vi "HEWH Check Ambient Temp.vi"(7 "Water Heater Type":T1, 8 "error in (no error)":errorcluster, 11 "UEF Calculated Values Input":T2 {"Data Indexes"."15 sec after Draw Index" format="%#.2f"; "Data Indexes"."15 sec after Draw Timestamp" format="%#.2f"; "Data Indexes"."Test Start Timestamp" format="%.2f"; "Data Indexes"."Test End Timestamp" format="%.2f"; "Data Indexes"."T0 Timestamp" format="%.2f"; "Data Indexes"."Tsf Timestamp" format="%.2f"; "Data Indexes"."Tsu0 Timestamp" format="%.2f"; "Data Indexes"."Tmax1 Timestamp" format="%.2f"; "Data Indexes"."Draw Index Timestamp" format="%#.2f"; "Data Indexes"."Non-Draw Timestamp" format="%#.2f"; "Data Indexes"."Heating Timestamp" format="%#.2f"; "Data Indexes"."Start Energy (BTU-Gas)" format="%.6f"; "Data Indexes"."Start Watt Hours" format="%.6f"; "Static Data"."V - Volume of Wh (True)" format="%.5f"; "Static Data"."T-Ambinet Nominal (°F)" format="%.5f"; "Static Data"."T-Inlet Setpoint (°F)" format="%.5f"; "Static Data"."T-Wh Setpoint (°F)" format="%.5f"; "Sampled Data"."Qe (Wh)" format="%.5f"; "Sampled Data"."Tau stby2 (hr)" format="%.5f"; "Sampled Data"."Tastby2 (°F)" format="%.5f"; "Sampled Data"."Qf (BTU)" format="%.5f"; "Sampled Data"."Qe (BTU)" format="%.5f"; "Sampled Data"."Tmax1 (°F)" format="%.5f"; "Sampled Data"."T0 (°F)" format="%.5f"; "Sampled Data"."Qr (BTU)" format="%.5f"; "Sampled Data"."T 24(°F)" format="%.5f"; "Sampled Data"."T astby(°F)" format="%.5f"; "Sampled Data"."T tstby(°F)" format="%.5f"; "Sampled Data"."T su0(°F)" format="%.5f"; "Sampled Data"."T suf(°F)" format="%.5f"; "Sampled Data"."Tau stby_1 (hr)" format="%.5f"; "Sampled Data"."Qsuf (BTU)" format="%.5f"; "Sampled Data"."Qsu0 (BTU)" format="%.5f"; "Calculated Values"."Draw Bonus Volume (gal)" format="%.6f"; "Calculated Values"."Adjustment Factor" format="%.6f"; "Calculated Values"."T*avg_del(n-1)" format="%.6f"; "Calculated Values"."T*min(n-1)" format="%.6f"; "Calculated Values"."T*avg_del(n)" format="%.6f"; "Calculated Values"."Vn" format="%.6f"; "Calculated Values"."Qdm (BTU)" format="%.6f"; "Calculated Values"."QHWD (BTU)" format="%.6f"; "Calculated Values"."QHW (BTU)" format="%.6f"; "Calculated Values"."UEF" format="%.6f"; "Calculated Values"."QHW67 (BTU)" format="%.6f"; "Calculated Values"."Qda (BTU)" format="%.6f"; "Calculated Values"."Qd (BTU)" format="%.6f"; "Calculated Values"."Q (BTU)" format="%.6f"; "Calculated Values"."UA (BTU/(hr*F))" format="%.6f"; "Calculated Values"."Qhr (BTU/hr)" format="%.6f"; "Calculated Values"."Qstby (BTU)" format="%.6f"; "Calculated Values"."nu_r" format="%.6f"; "Calculated Values"."CpUEF (BTU/(lb*F))" format="%.6f"; "Calculated Values"."rho_nu (lb/gal)" format="%.6f"; "Calculated Values"."V1- Vol (Gal)" format="%.6f"; "Calculated Values"."M cluster mass removed (lb)" format="%.6f"; "Calculated Values"."Cp theoretical (BTU/(lbm °F))" format="%.6f"; "Calculated Values"."Tin1 - Mean Inlet 1st Cluster (°F)" format="%.6f"; "Calculated Values"."Tdel1-Mean Outlet 1st Cluster(°F)" format="%.6f"; "Calculated Values"."Cp 24 (BTU/(lb*F))" format="%.6f"; "Calculated Values"."Cp standby (BTU/(lb*F))" format="%.6f"; "Calculated Values"."Cp2 (BTU/(lb*F))" format="%.6f"; "Calculated Values"."Cp1 (BTU/(lb*F))" format="%.6f"; "Calculated Values"."rho 24 (lb/gal)" format="%.6f"; "Calculated Values"."rho standby (lb/gal)" format="%.6f"; "Calculated Values"."rho 2 (lb/gal)" format="%.6f"; "Calculated Values"."Density of cold water All (lbm/gal)" format="%#.3g"; "Calculated Values"."CpHW (BTU/(lbm °F))" format="%#.3g"; "Calculated Values"."Density of hot water All (lbm/gal)" format="%#.3g"; "Calculated Values"."Mass of water All (lbm)" format="%#.3f"}) -> (0 "error out":errorcluster, 3 "UEF Calculated Values Output":T2 {"Data Indexes"."15 sec after Draw Index" format="%#.2f"; "Data Indexes"."15 sec after Draw Timestamp" format="%#.2f"; "Data Indexes"."Test Start Timestamp" format="%.2f"; "Data Indexes"."Test End Timestamp" format="%.2f"; "Data Indexes"."T0 Timestamp" format="%.2f"; "Data Indexes"."Tsf Timestamp" format="%.2f"; "Data Indexes"."Tsu0 Timestamp" format="%.2f"; "Data Indexes"."Tmax1 Timestamp" format="%.2f"; "Data Indexes"."Draw Index Timestamp" format="%#.2f"; "Data Indexes"."Non-Draw Timestamp" format="%#.2f"; "Data Indexes"."Heating Timestamp" format="%#.2f"; "Data Indexes"."Start Energy (BTU-Gas)" format="%.6f"; "Data Indexes"."Start Watt Hours" format="%.6f"; "Static Data"."V - Volume of Wh (True)" format="%.5f"; "Static Data"."T-Ambinet Nominal (°F)" format="%.5f"; "Static Data"."T-Inlet Setpoint (°F)" format="%.5f"; "Static Data"."T-Wh Setpoint (°F)" format="%.5f"; "Sampled Data"."Qe (Wh)" format="%.5f"; "Sampled Data"."Tau stby2 (hr)" format="%.5f"; "Sampled Data"."Tastby2 (°F)" format="%.5f"; "Sampled Data"."Qf (BTU)" format="%.5f"; "Sampled Data"."Qe (BTU)" format="%.5f"; "Sampled Data"."Tmax1 (°F)" format="%.5f"; "Sampled Data"."T0 (°F)" format="%.5f"; "Sampled Data"."Qr (BTU)" format="%.5f"; "Sampled Data"."T 24(°F)" format="%.5f"; "Sampled Data"."T astby(°F)" format="%.5f"; "Sampled Data"."T tstby(°F)" format="%.5f"; "Sampled Data"."T su0(°F)" format="%.5f"; "Sampled Data"."T suf(°F)" format="%.5f"; "Sampled Data"."Tau stby_1 (hr)" format="%.5f"; "Sampled Data"."Qsuf (BTU)" format="%.5f"; "Sampled Data"."Qsu0 (BTU)" format="%.5f"; "Calculated Values"."Draw Bonus Volume (gal)" format="%.6f"; "Calculated Values"."Adjustment Factor" format="%.6f"; "Calculated Values"."T*avg_del(n-1)" format="%.6f"; "Calculated Values"."T*min(n-1)" format="%.6f"; "Calculated Values"."T*avg_del(n)" format="%.6f"; "Calculated Values"."Vn" format="%.6f"; "Calculated Values"."Qdm (BTU)" format="%.6f"; "Calculated Values"."QHWD (BTU)" format="%.6f"; "Calculated Values"."QHW (BTU)" format="%.6f"; "Calculated Values"."UEF" format="%.6f"; "Calculated Values"."QHW67 (BTU)" format="%.6f"; "Calculated Values"."Qda (BTU)" format="%.6f"; "Calculated Values"."Qd (BTU)" format="%.6f"; "Calculated Values"."Q (BTU)" format="%.6f"; "Calculated Values"."UA (BTU/(hr*F))" format="%.6f"; "Calculated Values"."Qhr (BTU/hr)" format="%.6f"; "Calculated Values"."Qstby (BTU)" format="%.6f"; "Calculated Values"."nu_r" format="%.6f"; "Calculated Values"."CpUEF (BTU/(lb*F))" format="%.6f"; "Calculated Values"."rho_nu (lb/gal)" format="%.6f"; "Calculated Values"."V1- Vol (Gal)" format="%.6f"; "Calculated Values"."M cluster mass removed (lb)" format="%.6f"; "Calculated Values"."Cp theoretical (BTU/(lbm °F))" format="%.6f"; "Calculated Values"."Tin1 - Mean Inlet 1st Cluster (°F)" format="%.6f"; "Calculated Values"."Tdel1-Mean Outlet 1st Cluster(°F)" format="%.6f"; "Calculated Values"."Cp 24 (BTU/(lb*F))" format="%.6f"; "Calculated Values"."Cp standby (BTU/(lb*F))" format="%.6f"; "Calculated Values"."Cp2 (BTU/(lb*F))" format="%.6f"; "Calculated Values"."Cp1 (BTU/(lb*F))" format="%.6f"; "Calculated Values"."rho 24 (lb/gal)" format="%.6f"; "Calculated Values"."rho standby (lb/gal)" format="%.6f"; "Calculated Values"."rho 2 (lb/gal)" format="%.6f"; "Calculated Values"."Density of cold water All (lbm/gal)" format="%#.3g"; "Calculated Values"."CpHW (BTU/(lbm °F))" format="%#.3g"; "Calculated Values"."Density of hot water All (lbm/gal)" format="%#.3g"; "Calculated Values"."Mass of water All (lbm)" format="%#.3f"})   [LabVIEW 2023]
uses:
  Type Definitions/UEF Constants.ctl
  Type Definitions/HEWH Draw Stats.ctl
  Type Definitions/HEWH FHR Draw Type.ctl
  Type Definitions/FHR Bins.ctl
  Type Definitions/HEWH Meter Type.ctl
  Type Definitions/HEWH Water Heater Type.ctl
panel:
  # "FHR"
  # "FHR"
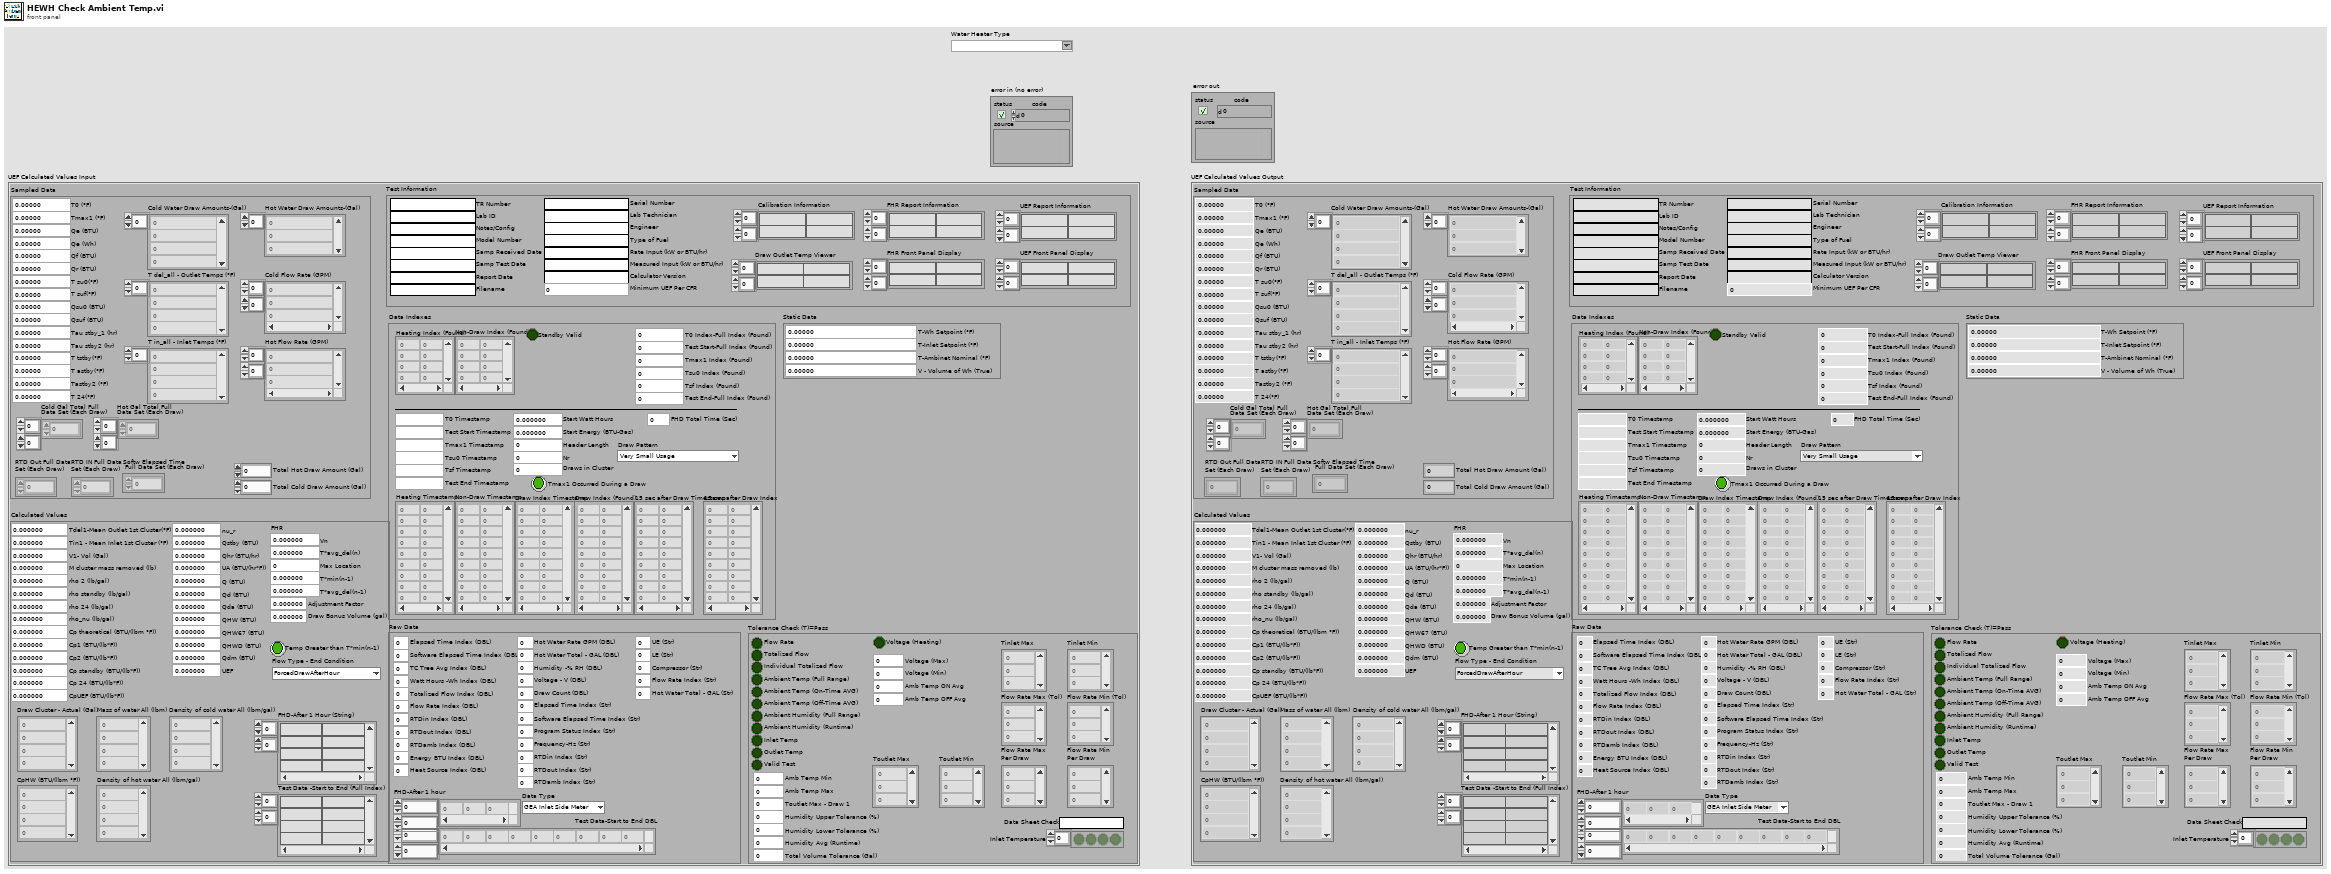
[diagram p1: front panel]
types:
  T1 = typedef "HEWH Water Heater Type.ctl" = string
  T2 = typedef "UEF Constants.ctl" = cluster{"Calculated Values":T3, "Sampled Data":cluster{"Cold Water Draw Amounts-(Gal)":dbl[], "T del_all - Outlet Temps (°F)":dbl[], "T in_all - Inlet Temps (°F)":dbl[], "Qsu0 (BTU)":dbl, "Qsuf (BTU)":dbl, "Tau stby_1 (hr)":dbl, "T suf(°F)":dbl, "T su0(°F)":dbl, "T tstby(°F)":dbl, "T astby(°F)":dbl, "T 24(°F)":dbl, "Qr (BTU)":dbl, "T0 (°F)":dbl, "Tmax1 (°F)":dbl, "Qe (BTU)":dbl, "Qf (BTU)":dbl, "Tastby2 (°F)":dbl, "RTD Out Full Data\nSet (Each Draw)":dbl[][], "RTD IN Full Data\nSet (Each Draw)":dbl[][], "Tau stby2 (hr)":dbl, "Hot Water Draw Amounts-(Gal)":dbl[], "Cold Flow Rate (GPM)":dbl[][], "Hot Flow Rate (GPM)":dbl[][], "Softw Elapsed Time\n Full Data Set (Each Draw)":dbl[][], "Cold Gal Total Full\nData Set (Each Draw)":dbl[][], "Total Hot Draw Amount (Gal) ":dbl, "Total Cold Draw Amount (Gal)":dbl, "Qe (Wh)":dbl, "Hot Gal Total Full\nData Set (Each Draw)":dbl[][]}, "Static Data":cluster{"T-Wh Setpoint (°F)":dbl, "T-Inlet Setpoint (°F)":dbl, "T-Ambinet Nominal (°F)":dbl, "V - Volume of Wh (True)":dbl}, "Data Indexes":cluster{"Test Start-Full Index (Found)":i32, "Header Length":i32, "Draw Index (Found)":i32[][], "Nr":i32, "Start Watt Hours":dbl, "Tsu0 Index (Found)":i32, "Tsf Index (Found)":i32, "Start Energy (BTU-Gas)":dbl, "Draws in Cluster":i32, "T0 Index-Full Index (Found)":i32, "Non-Draw Index (Found)":i32[][], "Tmax1 Index (Found)":i32, "Test End-Full Index (Found)":i32, "Heating Index (Found)":i32[][], "Heating Timestamp":dbl[][], "Non-Draw Timestamp":dbl[][], "Draw Index Timestamp":dbl[][], "Tmax1 Timestamp":dbl, "Tsu0 Timestamp":dbl, "Tsf Timestamp":dbl, "T0 Timestamp":dbl, "Test End Timestamp":dbl, "Test Start Timestamp":dbl, "15 sec after Draw Timestamp":dbl[][], "15 sec after Draw Index":dbl[][], "Tmax1 Occurred During a Draw":bool, "FHD Total Time (Sec)":dbl, "Draw Pattern":T5, "Standby Valid":bool}, "Raw Data":cluster{"Elapsed Time Index (DBL)":i32, "Software Elapsed Time Index (DBL)":i32, "TC Tree Avg Index (DBL)":i32, "Watt Hours -Wh Index (DBL)":i32, "Energy BTU Index (DBL)":i32, "Totalized Flow Index (DBL)":i32, "Flow Rate Index (DBL)":i32, "Program Status Index (Str)":i32, "RTDin Index (DBL)":i32, "RTDout Index (DBL)":i32, "RTDamb Index (DBL)":i32, "Test Data-Start to End DBL":dbl[][], "Data Type":T6, "Heat Source Index (DBL)":i32, "Hot Water Rate GPM (DBL)":i32, "Hot Water Total - GAL (DBL)":i32, "FHD-After 1 hour":dbl[][], "Humidity -% RH (DBL)":i32, "Voltage - V (DBL)":i32, "Draw Count (DBL)":i32, "Elapsed Time Index (Str)":i32, "Software Elapsed Time Index (Str)":i32, "Frequency-Hz (Str)":i32, "RTDin Index (Str)":i32, "RTDout Index (Str)":i32, "RTDamb Index (Str)":i32, "UE (Str)":i32, "LE (Str)":i32, "Compressor (Str)":i32, "Flow Rate Index (Str)":i32, "Hot Water Total - GAL (Str)":i32}, "Tolerance Check (T)=Pass":cluster{"Flow Rate":bool, "Totalized Flow":bool, "Ambient Temp (Full Range)":bool, "Ambient Humidity (Full Range)":bool, "Inlet Temp":bool, "Outlet Temp":bool, "Valid Test":bool, "Individual Totalized Flow":bool, "Data Sheet Check":string, "Inlet Temperature":bool[], "Tinlet Max":dbl[], "Tinlet Min":dbl[], "Flow Rate Max (Tol)":dbl[], "Flow Rate Min (Tol)":dbl[], "Amb Temp Max":dbl, "Amb Temp Min":dbl, "Toutlet Max - Draw 1":dbl, "Humidity Upper Tolerance (%)":dbl, "Total Volume Tolerance (Gal)":dbl, "Humidity Lower Tolerance (%)":dbl, "Flow Rate Max\nPer Draw":dbl[], "Flow Rate Min\nPer Draw":dbl[], "Ambient Humidity (Runtime)":bool, "Humidity Avg (Runtime)":dbl, "Ambient Temp (On-Time AVG)":bool, "Ambient Temp (Off-Time AVG)":bool, "Amb Temp OFF Avg":dbl, "Amb Temp ON Avg":dbl, "Voltage (Heating)":bool, "Voltage (Min)":dbl, "Voltage (Max)":dbl, "Toutlet Max":dbl[], "Toutlet Min":dbl[]}, "Test Information":cluster{"TR Number":string, "Lab ID":string, "Notes/Config":string, "Model Number":string, "Serial Number":string, "Lab Technician":string, "Engineer":string, "Type of Fuel":string, "Samp Received Date":string, "Samp Test Date":string, "Report Date":string, "Rate Input (kW or BTU/hr)":string, "Measured Input (kW or BTU/hr)":string, "Filename":string, "Calibration Information":string[][], "Calculator Version":string, "Minimum UEF Per CFR":dbl, "UEF Report Information":string[][], "FHR Report Information":string[][], "FHR Front Panel Display":string[][], "UEF Front Panel Display":string[][], "Draw Outlet Temp Viewer":string[][]}}
  T3 = typedef "HEWH Draw Stats.ctl" = cluster{"Draw Cluster - Actual (Gal)":dbl[], "Mass of water All (lbm)":dbl[], "Density of hot water All (lbm/gal)":dbl[], "CpHW (BTU/(lbm °F))":dbl[], "rho 2 (lb/gal)":dbl, "rho standby (lb/gal)":dbl, "rho 24 (lb/gal)":dbl, "Cp1 (BTU/(lb*F))":dbl, "Cp2 (BTU/(lb*F))":dbl, "Cp standby (BTU/(lb*F))":dbl, "Cp 24 (BTU/(lb*F))":dbl, "nu_r":dbl, "Qstby (BTU)":dbl, "Qhr (BTU/hr)":dbl, "UA (BTU/(hr*F))":dbl, "Q (BTU)":dbl, "Qd (BTU)":dbl, "Qda (BTU)":dbl, "QHW67 (BTU)":dbl, "UEF":dbl, "Tdel1-Mean Outlet 1st Cluster(°F)":dbl, "Tin1 - Mean Inlet 1st Cluster (°F)":dbl, "Cp theoretical (BTU/(lbm °F))":dbl, "M cluster mass removed (lb)":dbl, "V1- Vol (Gal)":dbl, "Test Data -Start to End (Full Index)":string[][], "rho_nu (lb/gal)":dbl, "Density of cold water All (lbm/gal)":dbl[], "CpUEF (BTU/(lb*F))":dbl, "QHW (BTU)":dbl, "QHWD (BTU)":dbl, "Qdm (BTU)":dbl, "FHD-After 1 Hour (String)":string[][], "Vn":dbl, "T*avg_del(n)":dbl, "Max Location":i32, "T*min(n-1)":dbl, "T*avg_del(n-1)":dbl, "Temp Greater than T*min(n-1)":bool, "Adjustment Factor":dbl, "Draw Bonus Volume (gal)":dbl, "Flow Type - End Condition":T4}
  T4 = typedef "HEWH FHR Draw Type.ctl" = enum16{"ForcedDrawAfterHour", "HeatingCutoffBeforeHour"}
  T5 = typedef "FHR Bins.ctl" = enum16{"Very Small Usage", "Low Usage", "Medium Usage", "High Usage", "Undefined"}
  T6 = typedef "HEWH Meter Type.ctl" = enum16{"GEA Inlet Side Meter", "GEA Outlet Side Meter", "CSA Inlet Side Meter"}
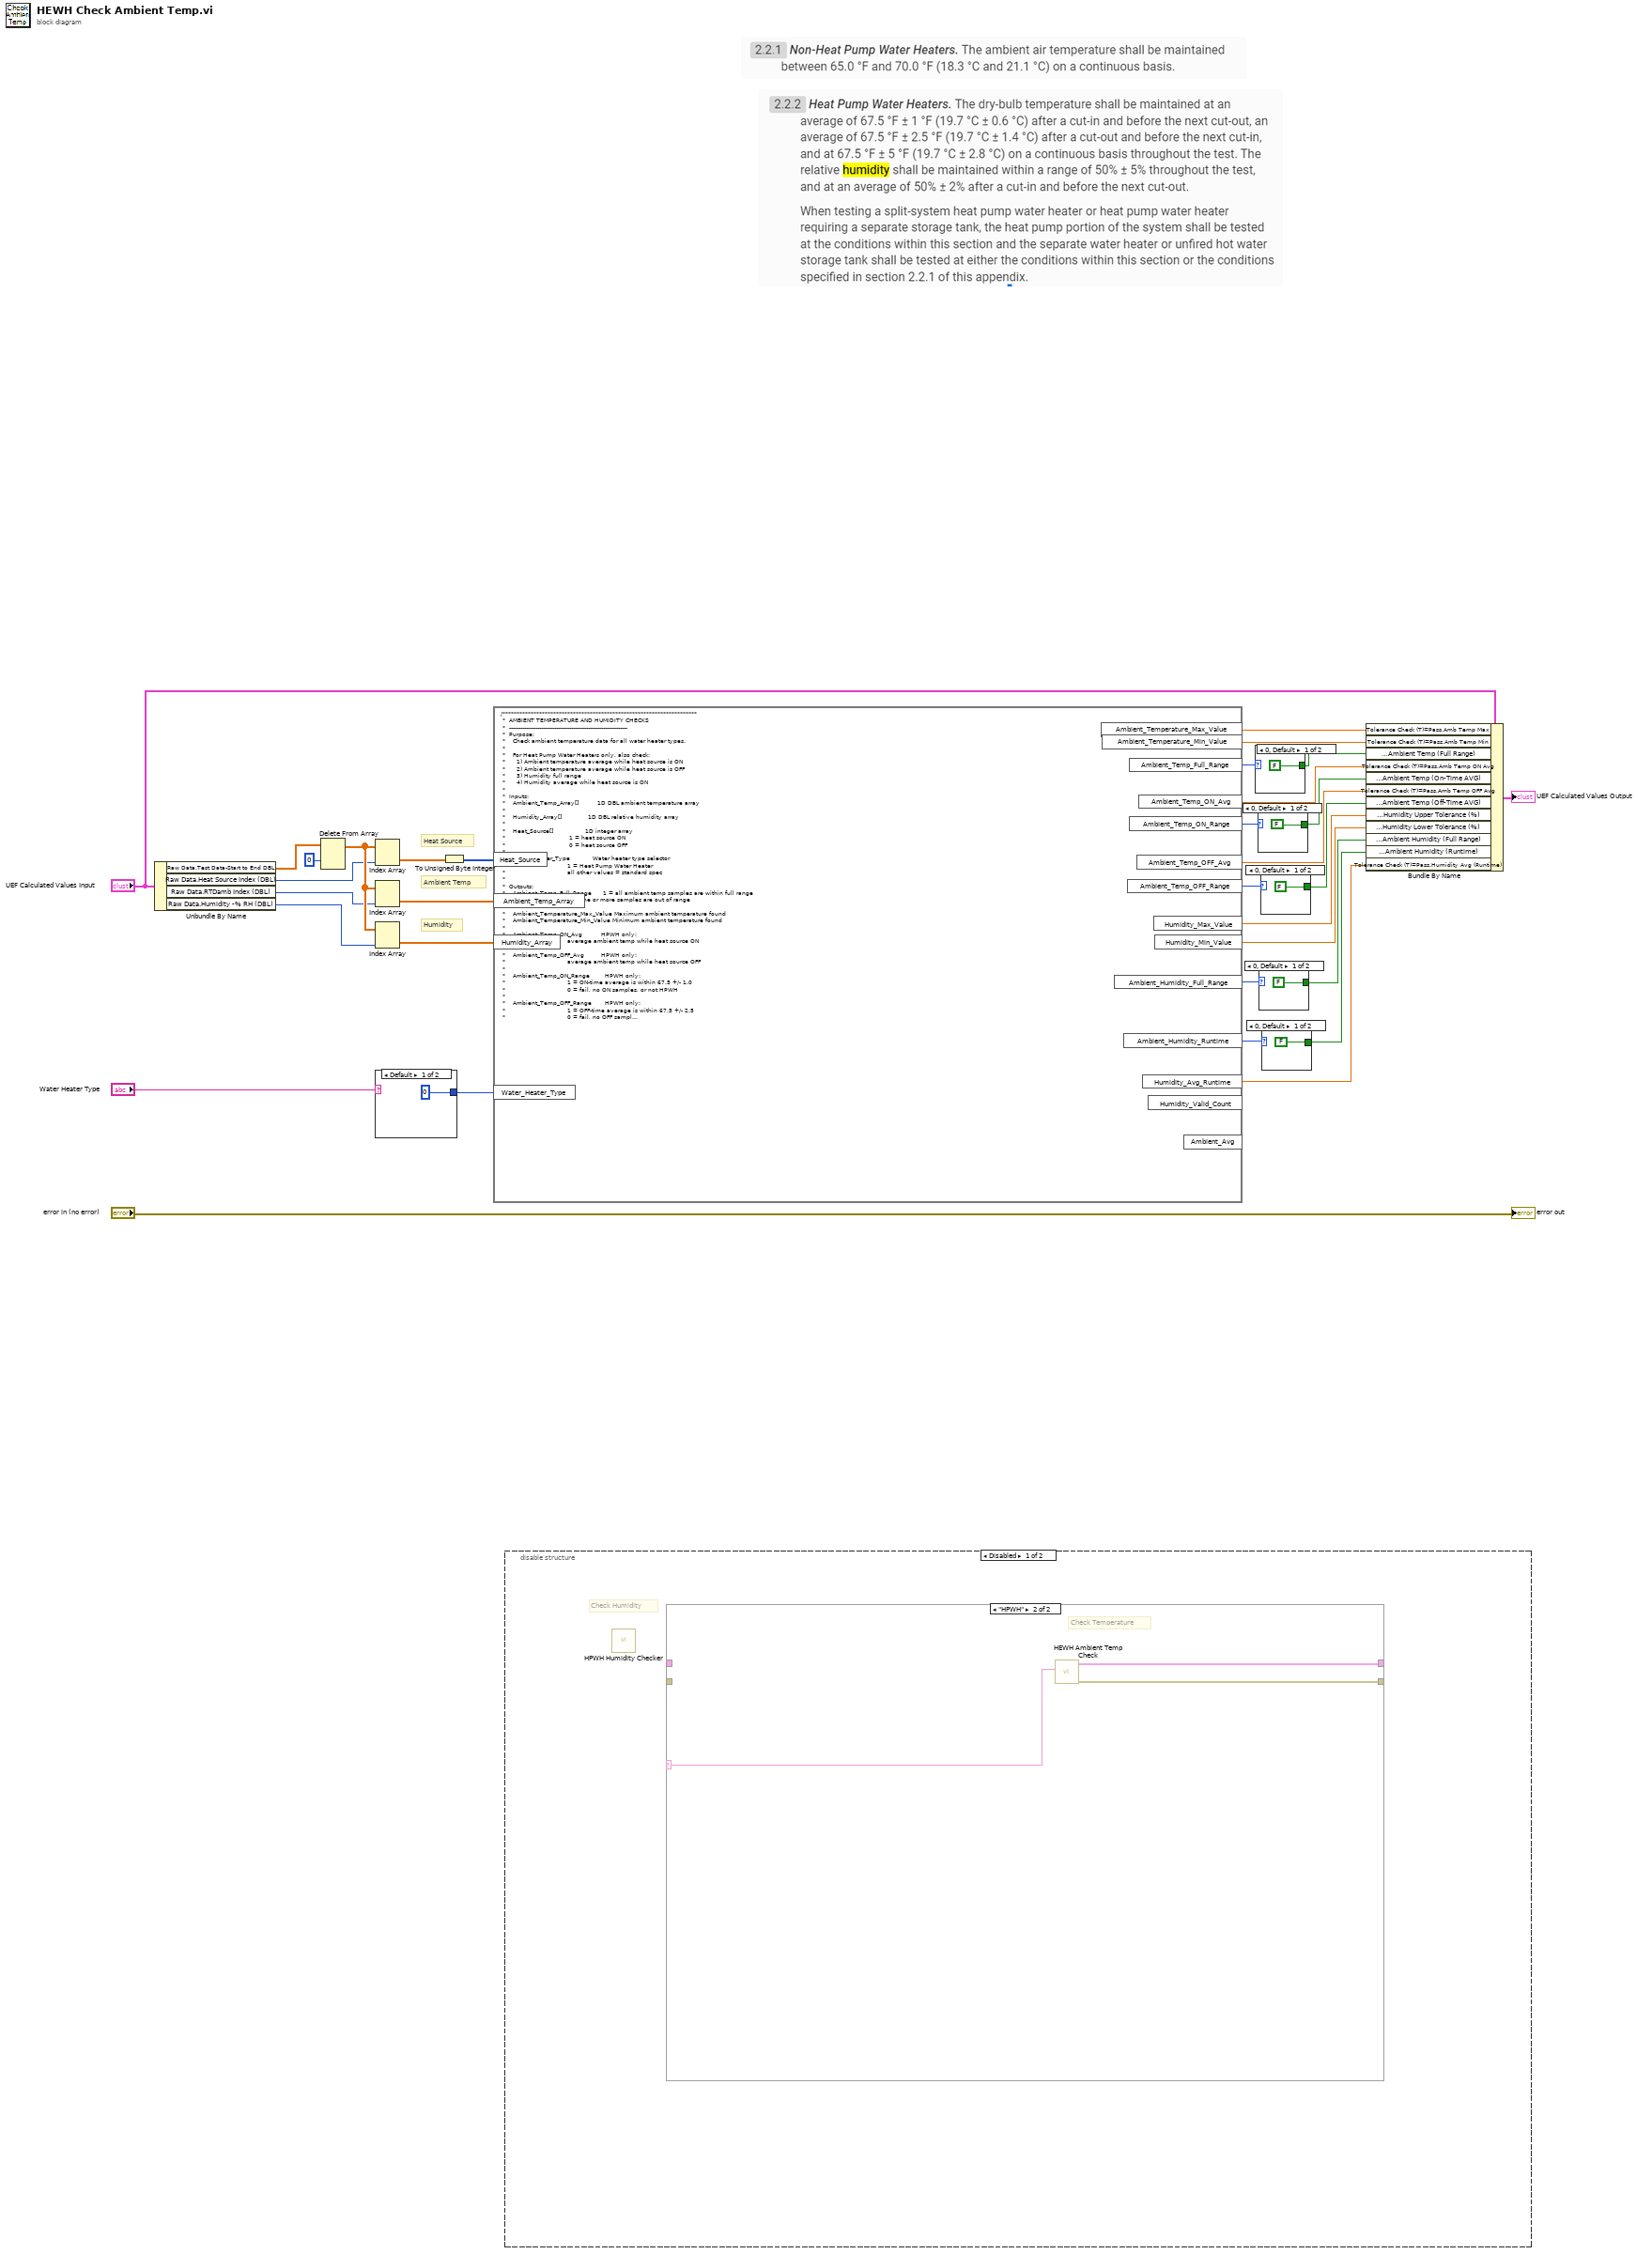
[diagram p0: block diagram]
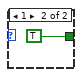
[diagram p2: hidden frame]
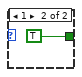
[diagram p3: hidden frame]
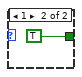
[diagram p4: hidden frame]
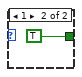
[diagram p5: hidden frame]
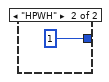
[diagram p6: hidden frame]
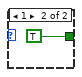
[diagram p7: hidden frame]
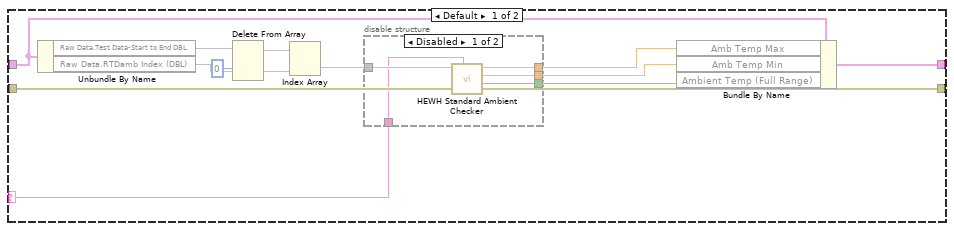
[diagram p8: hidden frame]
diagram:
  # "Humidity"
  # "Ambient Temp"
  # "Heat Source"
  n1 = Unbundle By Name("UEF Calculated Values Input") -> ("Raw Data.Test Data-Start to End DBL"=w9:dbl[][], "Raw Data.Heat Source Index (DBL)"=w7:i32, "Raw Data.RTDamb Index (DBL)"=w8:i32, "Raw Data.Humidity -% RH (DBL)"=w19:i32)
  n2 = Delete From Array(array=w9, index (row)=0) -> (array with subset deleted=w18:dbl[][])  [unwired: 2 in, 1 out]
  n3 = Index Array(array=w18, index (col)=w7) -> (element=w10:dbl[])  [unwired: 1 in]
  n4 = Index Array(array=w18, index (col)=w8) -> (element=w13:dbl[])  [unwired: 1 in]
  n5 = Index Array(array=w18, index (col)=w19) -> (element=w1:dbl[])  [unwired: 1 in]
  n6 = case shown="Default" "Water Heater Type" {
    tunnel: [0 ("Water_Heater_Type") 1 ("Water_Heater_Type")] -> w11
    frame Default {
    }
    frame "HPWH" {
    }
  }
  n7 = To Unsigned Byte Integer(number=w10) -> (unsigned 8bit integer=w14:u8[])
  n8 = formula code="/*********************************************************************\n *  AMBIENT TEMPERATURE AND HUMIDITY CHECKS\n *  ---------------------------------------------------------------\n *  Purpose:\n *    Check ambient temperature data for all water heater types.\n *\n *    For Heat Pump Water Heaters only, also check:\n *      1) Ambient temperature average while heat source is ON\n *      2) Ambient temperature average while heat source is OFF\n *      3) Humidity full range\n *      4) Humidity average while heat source is ON\n *\n *  Inputs:\n *    Ambient_Temp_Array[]          1D DBL ambient temperature array\n *\n *    Humidity_Array[]              1D DBL relative humidity array\n *\n *    Heat_Source[]                 1D integer array\n *                                  1 = heat source ON\n *                                  0 = heat source OFF\n *\n *    Water_Heater_Type            Water heater type selector\n *                                 1 = Heat Pump Water Heater\n *                                 all other values = standard spec\n *\n *  Outputs:\n *    Ambient_Temp_Full_Range      1 = all ambient temp samples are within full range\n *                                 0 = one or more samples are out of range\n *\n *    Ambient_Temperature_Max_Value Maximum ambient temperature found\n *    Ambient_Temperature_Min_Value Minimum ambient temperature found\n *\n *    Ambient_Temp_ON_Avg          HPWH only:\n *                                 average ambient temp while heat source ON\n *\n *    Ambient_Temp_OFF_Avg         HPWH only:\n *                                 average ambient temp while heat source OFF\n *\n *    Ambient_Temp_ON_Range        HPWH only:\n *                                 1 = ON-time average is within 67.5 +/- 1.0\n *                                 0 = fail, no ON samples, or not HPWH\n *\n *    Ambient_Temp_OFF_Range       HPWH only:\n *                                 1 = OFF-time average is within 67.5 +/- 2.5\n *                                 0 = fail, no OFF samples, or not HPWH\n *\n *    Humidity_Max_Value           HPWH only:\n *                                 maximum humidity value found\n *\n *    Humidity_Min_Value           HPWH only:\n *                                 minimum humidity value found\n *\n *    Ambient_Humidity_Full_Range HPWH only:\n *                                 1 = full humidity array is within 50 +/- 5%\n *                                 0 = fail, empty array, or not HPWH\n *\n *    Humidity_Avg_Runtime         HPWH only:\n *                                 average humidity while heat source is ON\n *\n *    Ambient_Humidity_Runtime     HPWH only:\n *                                 1 = runtime humidity average is within 50 +/- 2%\n *                                 0 = fail, no ON samples, or not HPWH\n *\n *  Ambient Temperature Full Range Logic:\n *    Heat Pump Water Heater:\n *      Lower = 62.5\n *      Upper = 72.5\n *\n *    All other water heater types:\n *      Lower = 65.0\n *      Upper = 70.0\n *\n *  HPWH Ambient ON/OFF Average Logic:\n *    ON-time average:\n *      Lower = 66.5\n *      Upper = 68.5\n *\n *    OFF-time average:\n *      Lower = 65.0\n *      Upper = 70.0\n *\n *  HPWH Humidity Logic:\n *    Full-range humidity:\n *      Lower = 45.0\n *      Upper = 55.0\n *\n *    Runtime average humidity:\n *      Lower = 48.0\n *      Upper = 52.0\n *********************************************************************/\n\n\n/* ---------------- Local variables -------------------------------- */\n\nint32 i;\n\nint32 N;\nint32 N_Heat;\nint32 Loop_N;\n\nint32 ON_Count;\nint32 OFF_Count;\n\nfloat Selected_Upper_Spec;\nfloat Selected_Lower_Spec;\n\nfloat ON_Upper_Spec;\nfloat ON_Lower_Spec;\n\nfloat OFF_Upper_Spec;\nfloat OFF_Lower_Spec;\n\nfloat Ambient_Value;\nfloat ON_Sum;\nfloat OFF_Sum;\n\nfloat Ambient_Sum;\nfloat Ambient_Avg;\n\n\n/* ---------------- Humidity local variables ------------------------ */\n\nint32 N_Humidity;\nint32 Humidity_Loop_N;\nint32 Humidity_ON_Count;\n\nfloat Humidity_Value;\n\nfloat Humidity_ON_Sum;\n\nfloat Humidity_Runtime_Upper_Spec;\nfloat Humidity_Runtime_Lower_Spec;\n\nfloat Humidity_Upper_Tolerance = 0.0;\nfloat Humidity_Lower_Tolerance = 0.0;\n\n\n/* ---------------- Default outputs -------------------------------- */\n\nint32 Ambient_Temp_Full_Range = 0;\n\nAmbient_Temperature_Max_Value = 0.0;\nAmbient_Temperature_Min_Value = 0.0;\n\nAmbient_Temp_ON_Avg = 0.0;\nAmbient_Temp_OFF_Avg = 0.0;\n\nint32 Ambient_Temp_ON_Range = 0;\nint32 Ambient_Temp_OFF_Range = 0;\n\nHumidity_Max_Value = 0.0;\nHumidity_Min_Value = 0.0;\n\nint32 Ambient_Humidity_Full_Range = 0;\nint32 Ambient_Humidity_Runtime = 0;\n\nHumidity_Avg_Runtime = 0.0;\n\n\n/* ---------------- Default local values ---------------------------- */\n\nON_Count = 0;\nOFF_Count = 0;\n\nON_Sum = 0.0;\nOFF_Sum = 0.0;\n\nHumidity_ON_Count = 0;\nHumidity_ON_Sum = 0.0;\n\nHumidity_Max_Value = 0.0;\nHumidity_Min_Value = 0.0;\n int32 Humidity_Valid_Count;\n\n\n/* ---------------- Select full-range ambient specification --------- */\n\nif (Water_Heater_Type == 1)\n{\n    /*\n     * Heat Pump Water Heater full-range ambient specification.\n     */\n\n    Selected_Upper_Spec = 67.5 + 5.0;\n    Selected_Lower_Spec = 67.5 - 5.0;\n}\nelse\n{\n    /*\n     * Standard full-range ambient specification for all other types.\n     */\n\n    Selected_Upper_Spec = 70.0;\n    Selected_Lower_Spec = 65.0;\n}\n\n\n/* ---------------- HPWH ambient ON/OFF average specifications ------- */\n\nON_Upper_Spec = 67.5 + 1.0;\nON_Lower_Spec = 67.5 - 1.0;\n\nOFF_Upper_Spec = 67.5 + 2.5;\nOFF_Lower_Spec = 67.5 - 2.5;\n\n\n/* ---------------- HPWH humidity specifications -------------------- */\n\nHumidity_Upper_Tolerance = 50.0 + 5.0;\nHumidity_Lower_Tolerance = 50.0 - 5.0;\n\nHumidity_Runtime_Upper_Spec = 50.0 + 2.0;\nHumidity_Runtime_Lower_Spec = 50.0 - 2.0;\n\n\n/* ---------------- Get array lengths ------------------------------- */\n\nN = sizeOfDim(Ambient_Temp_Array, 0);\nN_Heat = sizeOfDim(Heat_Source, 0);\nN_Humidity = sizeOfDim(Humidity_Array, 0);\n\n\n/* ---------------- Evaluate ambient temperature data --------------- */\n\nif (N > 0)\n{\n    /*\n     * Initialize ambient min, max, and average sum.\n     */\n\n    Ambient_Temperature_Max_Value = Ambient_Temp_Array[0];\n    Ambient_Temperature_Min_Value = Ambient_Temp_Array[0];\n    Ambient_Sum = Ambient_Temp_Array[0];\n\n    /*\n     * Loop through the remaining ambient array values and find\n     * the maximum, minimum, and total ambient temperature values.\n     */\n\n    for (i = 1; i < N; i++)\n    {\n        Ambient_Value = Ambient_Temp_Array[i];\n\n        Ambient_Sum += Ambient_Value;\n\n\n        if (Ambient_Value > Ambient_Temperature_Max_Value)\n        {\n            Ambient_Temperature_Max_Value = Ambient_Value;\n        }\n\n\n        if (Ambient_Value < Ambient_Temperature_Min_Value)\n        {\n            Ambient_Temperature_Min_Value = Ambient_Value;\n        }\n    }\n\n\n    /*\n     * Calculate full-test ambient average.\n     */\n\n    Ambient_Avg = Ambient_Sum / N;\n\n\n    /*\n     * Check ambient temperature compliance.\n     *\n     * HPWH:\n     *   Full array must stay within 67.5 +/- 5.0:\n     *   62.5 to 72.5 F\n     *\n     * Non-HPWH:\n     *   Average must stay within 67.5 +/- 2.5:\n     *   65.0 to 70.0 F\n     *\n     *   Full array maximum deviation must stay within 67.5 +/- 5.0:\n     *   62.5 to 72.5 F\n     */\n\n    if (Water_Heater_Type == 1)\n    {\n        /*\n         * Heat Pump Water Heater full ambient range check.\n         */\n\n        if (Ambient_Temperature_Max_Value <= Selected_Upper_Spec &&\n            Ambient_Temperature_Min_Value >= Selected_Lower_Spec)\n        {\n            Ambient_Temp_Full_Range = 1;\n        }\n        else\n        {\n            Ambient_Temp_Full_Range = 0;\n        }\n    }\n    else\n    {\n        /*\n         * Non-HPWH ambient average and max-deviation check.\n         */\n\n        if (Ambient_Avg >= Selected_Lower_Spec &&\n            Ambient_Avg <=  Selected_Upper_Spec &&\n            Ambient_Temperature_Max_Value <= 72.5 &&\n            Ambient_Temperature_Min_Value >= 62.5)\n        {\n            Ambient_Temp_Full_Range = 1;\n        }\n        else\n        {\n            Ambient_Temp_Full_Range = 0;\n        }\n    }\n\n\n    /*****************************************************************\n     * HPWH ONLY:\n     *   Ambient temperature ON/OFF average checks.\n     *****************************************************************/\n\n    if (Water_Heater_Type == 1)\n    {\n        /*\n         * Only run ON/OFF ambient checks if the Heat_Source array has data.\n         */\n\n        if (N_Heat > 0)\n        {\n            /*\n             * Use the smaller array length if Ambient_Temp_Array and\n             * Heat_Source are not the same size.\n             */\n\n            Loop_N = N;\n\n            if (N_Heat < Loop_N)\n            {\n                Loop_N = N_Heat;\n            }\n\n\n            /*\n             * Separate ambient temperature samples into ON-time and\n             * OFF-time groups.\n             */\n\n            for (i = 0; i < Loop_N; i++)\n            {\n                if (Heat_Source[i] == 1)\n                {\n                    ON_Sum += Ambient_Temp_Array[i];\n                    ON_Count += 1;\n                }\n                else if (Heat_Source[i] == 0)\n                {\n                    OFF_Sum += Ambient_Temp_Array[i];\n                    OFF_Count += 1;\n                }\n            }\n\n\n            /*\n             * Calculate ON-time ambient average and check tolerance.\n             */\n\n            if (ON_Count > 0)\n            {\n                Ambient_Temp_ON_Avg = ON_Sum / ON_Count;\n\n                if (Ambient_Temp_ON_Avg >= ON_Lower_Spec &&\n                    Ambient_Temp_ON_Avg <= ON_Upper_Spec)\n                {\n                    Ambient_Temp_ON_Range = 1;\n                }\n                else\n                {\n                    Ambient_Temp_ON_Range = 0;\n                }\n            }\n            else\n            {\n                Ambient_Temp_ON_Avg = 0.0;\n                Ambient_Temp_ON_Range = 0;\n            }\n\n\n            /*\n             * Calculate OFF-time ambient average and check tolerance.\n             */\n\n            if (OFF_Count > 0)\n            {\n                Ambient_Temp_OFF_Avg = OFF_Sum / OFF_Count;\n\n                if (Ambient_Temp_OFF_Avg >= OFF_Lower_Spec &&\n                    Ambient_Temp_OFF_Avg <= OFF_Upper_Spec)\n                {\n                    Ambient_Temp_OFF_Range = 1;\n                }\n                else\n                {\n                    Ambient_Temp_OFF_Range = 0;\n                }\n            }\n            else\n            {\n                Ambient_Temp_OFF_Avg = 0.0;\n                Ambient_Temp_OFF_Range = 0;\n            }\n        }\n\n\n        /*************************************************************\n         * HPWH ONLY:\n         *   Humidity full-range and runtime average checks.\n         *************************************************************/\n\n        if (N_Humidity > 0)\n        {\n            /*\n              * Initialize and find full-array humidity min and max.\n              * Ignore invalid humidity values <= 0.0.\n               */\n               \n                Humidity_Valid_Count = 0;\n                Humidity_Max_Value = 0.0;\n                Humidity_Min_Value = 0.0;\n\n                for (i = 0; i < N_Humidity; i++)\n                {\n                   Humidity_Value = Humidity_Array[i];\n\n                   if (Humidity_Value > 0.0)\n                    {\n                       if (Humidity_Valid_Count == 0)\n                          {\n                             Humidity_Max_Value = Humidity_Value;\n                             Humidity_Min_Value = Humidity_Value;\n                          }\n                       else\n                         {\n                           if (Humidity_Value > Humidity_Max_Value)\n                              {\n                                Humidity_Max_Value = Humidity_Value;\n                              }\n\n                           if (Humidity_Value < Humidity_Min_Value)\n                              {\n                                Humidity_Min_Value = Humidity_Value;\n                              }\n                          }\n\n                          Humidity_Valid_Count += 1;\n                    }\n                }\n\n            /*\n             * Check full humidity range: 50 +/- 5%.\n             */\n\n            if (Humidity_Valid_Count > 0)\n            {\n                if (Humidity_Max_Value <= Humidity_Upper_Tolerance &&\n                    Humidity_Min_Value >= Humidity_Lower_Tolerance)\n               {\n                    Ambient_Humidity_Full_Range = 1;\n               }\n                else\n                {\n                    Ambient_Humidity_Full_Range = 0;\n                }\n            }\n            else\n            {\n                Humidity_Max_Value = 0.0;\n                Humidity_Min_Value = 0.0;\n                Ambient_Humidity_Full_Range = 0;\n            }\n\n\n            /*\n             * Runtime humidity average.\n             * Only use humidity samples where Heat_Source == 1.\n             */\n\n            if (N_Heat > 0)\n            {\n                Humidity_Loop_N = N_Humidity;\n\n                if (N_Heat < Humidity_Loop_N)\n                {\n                    Humidity_Loop_N = N_Heat;\n                }\n\n\n                for (i = 0; i < Humidity_Loop_N; i++)\n                {\n                    if (Heat_Source[i] == 1 && Humidity_Array[i]>0.0)\n                    {\n                        Humidity_ON_Sum += Humidity_Array[i];\n                        Humidity_ON_Count += 1;\n                    }\n                }\n\n\n                /*\n                 * Calculate runtime humidity average and check\n                 * tolerance: 50 +/- 2%.\n                 */\n\n                if (Humidity_ON_Count > 0)\n                {\n                    Humidity_Avg_Runtime = Humidity_ON_Sum / Humidity_ON_Count;\n\n                    if (Humidity_Avg_Runtime >= Humidity_Runtime_Lower_Spec &&\n                        Humidity_Avg_Runtime <= Humidity_Runtime_Upper_Spec)\n                    {\n                        Ambient_Humidity_Runtime = 1;\n                    }\n                    else\n                    {\n                        Ambient_Humidity_Runtime = 0;\n                    }\n                }\n                else\n                {\n                    Humidity_Avg_Runtime = 0.0;\n                    Ambient_Humidity_Runtime = 0;\n                }\n            }\n        }\n    }\n}\nelse\n{\n    /*\n     * Empty ambient array fault.\n     */\n\n    Ambient_Temp_Full_Range = 0;\n\n    Ambient_Temperature_Max_Value = 0.0;\n    Ambient_Temperature_Min_Value = 0.0;\n\n    Ambient_Temp_ON_Avg = 0.0;\n    Ambient_Temp_OFF_Avg = 0.0;\n\n    Ambient_Temp_ON_Range = 0;\n    Ambient_Temp_OFF_Range = 0;\n\n    Humidity_Max_Value = 0.0;\n    Humidity_Min_Value = 0.0;\n\n    Ambient_Humidity_Full_Range = 0;\n    Ambient_Humidity_Runtime = 0;\n\n    Humidity_Avg_Runtime = 0.0;\n}"("Ambient_Temp_Array"=w13, "Water_Heater_Type"=w11, "Heat_Source"=w14, "Humidity_Array"=w1) -> ("Ambient_Temp_Full_Range"=w12:i32, "Ambient_Temperature_Max_Value"=w16:dbl, "Ambient_Temperature_Min_Value"=w17:dbl, "Ambient_Temp_ON_Avg"=w20:dbl, "Ambient_Temp_OFF_Avg"=w21:dbl, "Ambient_Temp_ON_Range"=w22:i32, "Ambient_Temp_OFF_Range"=w24:i32, "Humidity_Max_Value"=w26:dbl, "Humidity_Min_Value"=w27:dbl, "Ambient_Humidity_Full_Range"=w28:i32, "Ambient_Humidity_Runtime"=w30:i32, "Humidity_Avg_Runtime"=w32:dbl)  [unwired: 2 out]
  n9 = disable-structure shown="Disabled" {
    frame Disabled {
      # "Check Humidity"
      n10 = call "HPWH Humidity Checker.vi"() -> ()  [unwired: 10 in, 2 out]
      n11 = case shown="\"HPWH\"" {
        selector: _ -> [w35 w52]
        tunnel: [w46 w53] -> _
        tunnel: _ -> [w40 _]
        tunnel: _ -> [w41 _]
        tunnel: [w41 w54] -> _
        frame Default {
          n12 = Unbundle By Name(w40) -> ("Raw Data.Test Data-Start to End DBL"=w43, "Raw Data.RTDamb Index (DBL)"=w44)
          n13 = Delete From Array(array=w43, index (row)=0) -> (array with subset deleted=w45)  [unwired: 2 in, 1 out]
          n14 = Index Array(array=w45, index (col)=w44) -> (element=w39)  [unwired: 1 in]
          n15 = disable-structure shown="Disabled" {
            disable-tunnel: w39 -> [w51 _]
            disable-tunnel: [w50 _] -> w38
            disable-tunnel: [w49 _] -> w37
            disable-tunnel: [w48 _] -> w36
            disable-tunnel: w35 -> [w47 _]
            frame Disabled {
              n16 = call "HEWH Standard Ambient Checker.vi"("Water Heater Type"=w47, "Ambient_Temp_Array"=w51) -> ("Ambient Temp (Full Range)"=w48:bool, "Ambient Temperature Min Value"=w49:dbl, "Ambient Temperature Max Value"=w50:dbl)  [unwired: 7 in]
            }
            frame Enabled {
            }
          }
          n17 = Bundle By Name(cluster=w40, "Amb Temp Max"=w38, "Amb Temp Min"=w37, "Ambient Temp (Full Range)"=w36) -> (w46:cluster{})
        }
        frame "HPWH" {
          # "Check Temperature"
          n18 = call "HEWH Ambient Temp Check.vi"("Water Heater Type"=w52) -> ("error out"=w54:errorcluster, "UEF Calculated Values Output"=w53:T2)  [unwired: 9 in]
        }
      }
    }
    frame Enabled {
    }
  }
  n19 = case shown="0, Default" w12 {
    tunnel: [FALSE TRUE] -> w15
    frame 0, Default {
    }
    frame 1 {
    }
  }
  n20 = case shown="0, Default" w22 {
    tunnel: [FALSE TRUE] -> w23
    frame 0, Default {
    }
    frame 1 {
    }
  }
  n21 = case shown="0, Default" w28 {
    tunnel: [FALSE TRUE] -> w29
    frame 0, Default {
    }
    frame 1 {
    }
  }
  n22 = case shown="0, Default" w24 {
    tunnel: [FALSE TRUE] -> w25
    frame 0, Default {
    }
    frame 1 {
    }
  }
  n23 = case shown="0, Default" w30 {
    tunnel: [FALSE TRUE] -> w31
    frame 0, Default {
    }
    frame 1 {
    }
  }
  n24 = Bundle By Name(cluster="UEF Calculated Values Input", "Tolerance Check (T)=Pass.Amb Temp Max"=w16, "Tolerance Check (T)=Pass.Amb Temp Min"=w17, "Tolerance Check (T)=Pass.Ambient Temp (Full Range)"=w15, "Tolerance Check (T)=Pass.Amb Temp ON Avg"=w20, "Tolerance Check (T)=Pass.Ambient Temp (On-Time AVG)"=w23, "Tolerance Check (T)=Pass.Amb Temp OFF Avg"=w21, "Tolerance Check (T)=Pass.Ambient Temp (Off-Time AVG)"=w25, "Tolerance Check (T)=Pass.Humidity Upper Tolerance (%)"=w26, "Tolerance Check (T)=Pass.Humidity Lower Tolerance (%)"=w27, "Tolerance Check (T)=Pass.Ambient Humidity (Full Range)"=w29, "Tolerance Check (T)=Pass.Ambient Humidity (Runtime)"=w31, "Tolerance Check (T)=Pass.Humidity Avg (Runtime)"=w32) -> (→"UEF Calculated Values Output":T2)
  "error out" <- "error in (no error)"
